vi "Update Credit.vi"(8 "error in (no error)":errorcluster, 10 "Credito":dbl, 11 "UI Actor in":refnum<class "UI Actor.lvclass">) -> (0 "error out":errorcluster, 3 "UI Actor out":refnum<class "UI Actor.lvclass">)   [LabVIEW 2019, in "UI Actor.lvlib" / "UI Actor.lvclass"]
uses:
  UI Actor.lvclass
  UI Actor.lvclass/UI Actor.ctl
  Mensajes Messages/Update Message event Msg/Update Message event Msg.lvclass/Update Message event Msg.ctl
  <vilib>/ActorFramework/Message Enqueuer/Message Enqueuer.lvclass/Message Enqueuer.ctl
  <vilib>/ActorFramework/Message Enqueuer/Enqueue.vi
  Mensajes Messages/Update Message event Msg/Update Message event Msg.lvclass
  C:/Program Files/National Instruments/LabVIEW 2019/vi.lib/ActorFramework/Message/Message.lvclass
  <vilib>/ActorFramework/Message Priority Queue/Priority Enqueue.vi
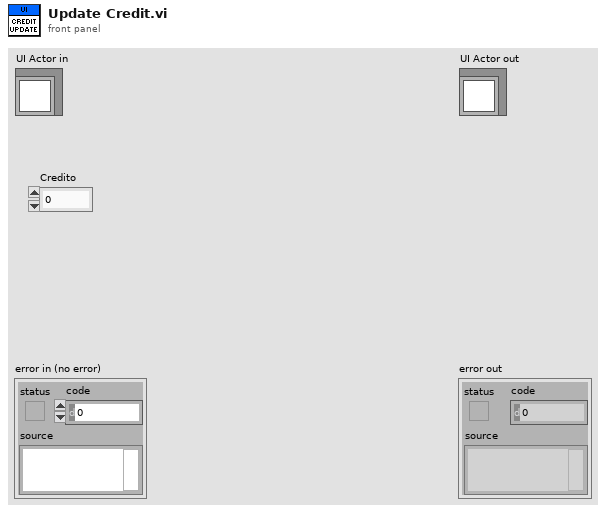
[diagram p1: front panel]
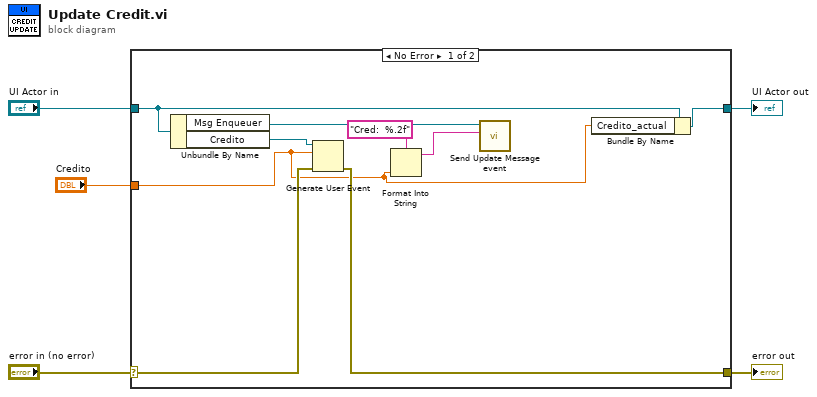
[diagram p0: block diagram]
diagram:
  n1 = case shown="No Error" "error in (no error)" {
    selector: "error in (no error)" -> [w13 w16]
    tunnel: [w12 w16] -> w4
    tunnel: [w7 w15] -> w2
    tunnel: "UI Actor in" -> [w8 w15]
    tunnel: "Credito" -> [w6 _]
    frame No Error {
      n2 = Unbundle By Name(w8) -> ("Msg Enqueuer"=w11:refnum<class "Message Enqueuer.lvclass">, "Credito"=w14:refnum<user-event>)
      n3 = Generate User Event(user event=w14, event data cluster=w6, error in=w13) -> (error out=w12:errorcluster)  [unwired: 1 in, 1 out]
      n4 = Format Into String(format string="Cred:  %.2f", w6) -> (resulting string=w9:string)  [unwired: 2 in, 1 out]
      n5 = call "Send Update Message event.vi"("Update Msg"=w9, "Message Enqueuer"=w11) -> ()  [unwired: 8 in, 2 out]
      n6 = Bundle By Name(cluster=w8, "Credito_actual"=w6) -> (w7:refnum<class "UI Actor.lvclass">)
    }
    frame Error {
    }
  }
  "error out" <- w4
  "UI Actor out" <- w2
